vi "SetPicture.vi"(8 "error in (no error)":errorcluster, 10 "Picture":picture, 11 "FolloWin in":refnum<class "FolloWin.lvclass">) -> (0 "error out":errorcluster, 3 "FolloWin out":refnum<class "FolloWin.lvclass">)   [LabVIEW 2023, in "FolloWin.lvclass"]
doc: "Sets picture to be shown in FolloWin window background (behind the text)"
uses:
  FolloWin.lvclass
  FolloWin.lvclass/FolloWin.ctl
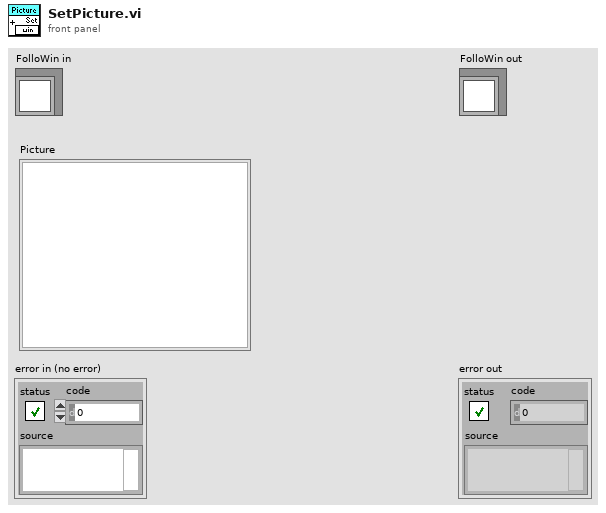
[diagram p1: front panel]
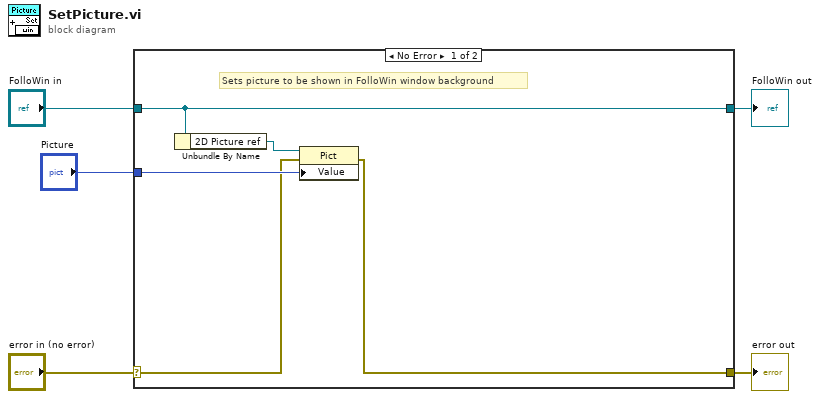
[diagram p0: block diagram]
diagram:
  n1 = case shown="No Error" "error in (no error)" {
    selector: "error in (no error)" -> [w7 w12]
    tunnel: [w6 w12] -> w4
    tunnel: [w10 w11] -> w2
    tunnel: "FolloWin in" -> [w10 w11]
    tunnel: "Picture" -> [w8 _]
    frame No Error {
      # "Sets picture to be shown in FolloWin window background"
      n2 = Unbundle By Name(w10) -> ("2D Picture ref"=w9:refnum<vi>)
      n3 = property on="Property Node" class="Pict"(reference=w9, error in=w7, "Value"=w8) -> (error out=w6:errorcluster)  [unwired: 1 out]
    }
    frame Error {
    }
  }
  "error out" <- w4
  "FolloWin out" <- w2
